vi "ESP32_Task_4.vi"() -> ()   [LabVIEW 2022 SP3]
doc: "This example performs writes and reads on a serial port, as directed by the user. You can press the Write and Read buttons, and change the Read Count, while the example is running.\n\nThe parameters set for the serial port must match the parameters of the connected instrument or device. In this example, the Read Count parameter specifies the number of bytes that the serial port reads. If there were more bytes at the port than the specified number, those bytes would not be read. If there were less bytes at the port than the specified number, you would receive a timeout error.\n\nThis example expands upon the flow control options for XON and XOFF, allowing the user to choose those control characters. Also, the user can enable or disable a termination character. Some devices require a termination character in order to identify the end of command strings. Some devices send a termination character to signify the end of data to be read. This example shows how you can end the Read operation once a termination character is detected in the buffer and/or append a termination character at the end of the Write data."
uses:
  Serial - Settings.ctl
  Serial - XON-XOFF Characters.ctl
  Serial - ASCII Characters.ctl
  ESP32-PSOC-State Machine.ctl
  <vilib>/Math Plots/2D Math Plots/2D Compass/2D Compass XCtrl/2D Compass.xctl
  <vilib>/Instr/_visa.llb/VISA Flush IO Buffer Mask.ctl
  <vilib>/Instr/_visa.llb/VISA Configure Serial Port (Instr).vi
  <vilib>/Math Plots/2D Math Plots/2D Compass/2D Compass Datatype/Public/Plot Helper (Vector).vi
  <vilib>/Math Plots/2D Math Plots/2D Compass/2D Compass Datatype/2D Compass Datatype.lvclass
panel:
  out "number 2":dbl
  out "number":dbl
  out "String":string
  out "XY Graph":cluster{"X":dbl, "Y":dbl}[](graph)
  out "2D Compass":refnum<class "2D Plot Datatype.lvclass">[](xcontrol)
  in  "Difficulty":T1
  out "error":bool
  out "Connected":bool
  out "Serial Settings:Number of Bytes at Serial Port":u32
  out "Response 2":string
  in  "Toggle LED":bool
  in  "Enum":T2
  in  "Termination Character":u8=10 format="%.0x"
  in  "End Write on Termination Character?":bool=TRUE
  in  "Stop":bool
  out "Read Count":u32=1000
  out "Response":string
  in  "XON/XOFF Characters":T3={"XON"=enum."DC1", "XOFF"=enum."DC3"}
  in  "Serial Settings":T5={"baud rate"=115200, "data bits"=8, "parity"=enum."None", "stop bits"=10, "flow control"=0} {"flow control" items=["None"=0, "XON/XOFF"=1, "RTS/CTS"=2, "DTR/DSR"=4]; "stop bits" items=["1.0"=10, "1.5"=15, "2.0"=20]; "data bits" min=5 max=8 step=1; "baud rate" items=["75"=75, "110"=110, "134"=134, "150"=150, "300"=300, "600"=600, "1200"=1200, "1800"=1800, "2400"=2400, "4800"=4800, "7200"=7200, "9600"=9600, "14400"=14400, "19200"=19200, "28800"=28800, "38400"=38400, "56000"=56000, "57600"=57600, "115200"=115200, "128000"=128000, "230400"=230400]}
  in  "End Read on Termination Character?":bool=TRUE
  in  "VISA resource name":refnum<visa-resource-name>="COM4"
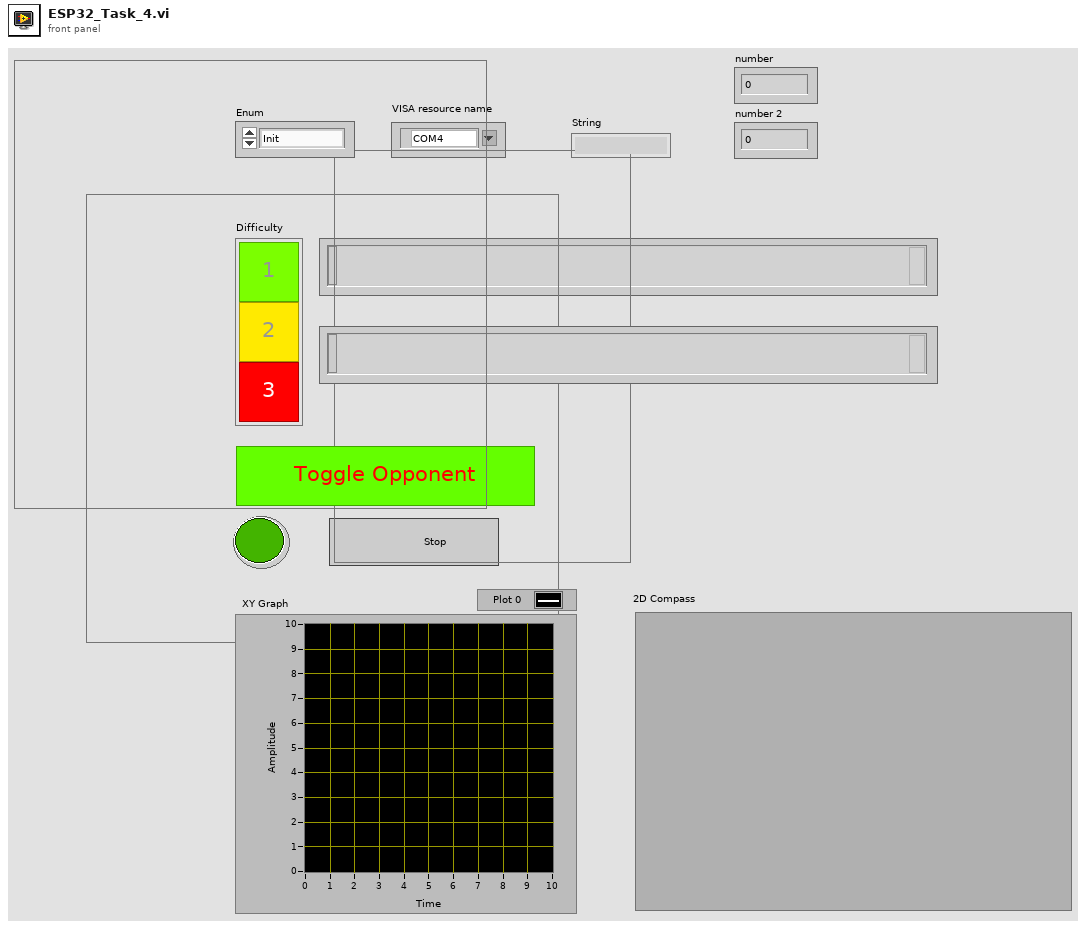
[diagram p1: front panel]
types:
  T1 = cluster{"Command A":bool, "Command B":bool, "Command C":bool}
  T2 = typedef "ESP32-PSOC-State Machine.ctl" = enum8{"Init", "Connect", "idle", "send", "wait", "receive", "que", "error", "exit"}
  T3 = typedef "Serial - XON-XOFF Characters.ctl" = cluster{"XON":T4, "XOFF":T4}
  T4 = typedef "Serial - ASCII Characters.ctl" = enum16{"NUL", "SOH", "STX", "ETX", "EOT", "ENQ", "ACK", "BEL", "BS", "HT", "LF", "VT", "FF", "CR", "SO", "SI", "DLE", "DC1", "DC2", "DC3", "DC4", "NAK", "SYN", "ETB", "CAN", "EM", "SUB", "ESC", "FS", "GS", "RS", "US", "SP", "!", "\"", "#", "$", "%", "&", "'", "(", ")", "*", "+", ",", "- (-)", ".", "/", "0", "1", "2", "3", "4", "5", "6", "7", "8", "9", ":", ";", "<", "=", ">", "?", "@", "A", "B", "C", "D", "E", "F", "G", "H", "I", "J", "K", "L", "M", "N", "O", "P", "Q", "R", "S", "T", "U", "V", "W", "X", "Y", "Z", "[", "\\", "]", "^", "_", "`", "a", "b", "c", "d", "e", "f", "g", "h", "i", "j", "k", "l", "m", "n", "o", "p", "q", "r", "s", "t", "u", "v", "w", "x", "y", "z", "{", "|", "}", "~"}
  T5 = typedef "Serial - Settings.ctl" = cluster{"baud rate":u32, "data bits":u16, "parity":enum16{"None", "Odd", "Even", "Mark", "Space"}, "stop bits":u16, "flow control":u16}
  T6 = typedef "VISA Flush IO Buffer Mask.ctl" = u16
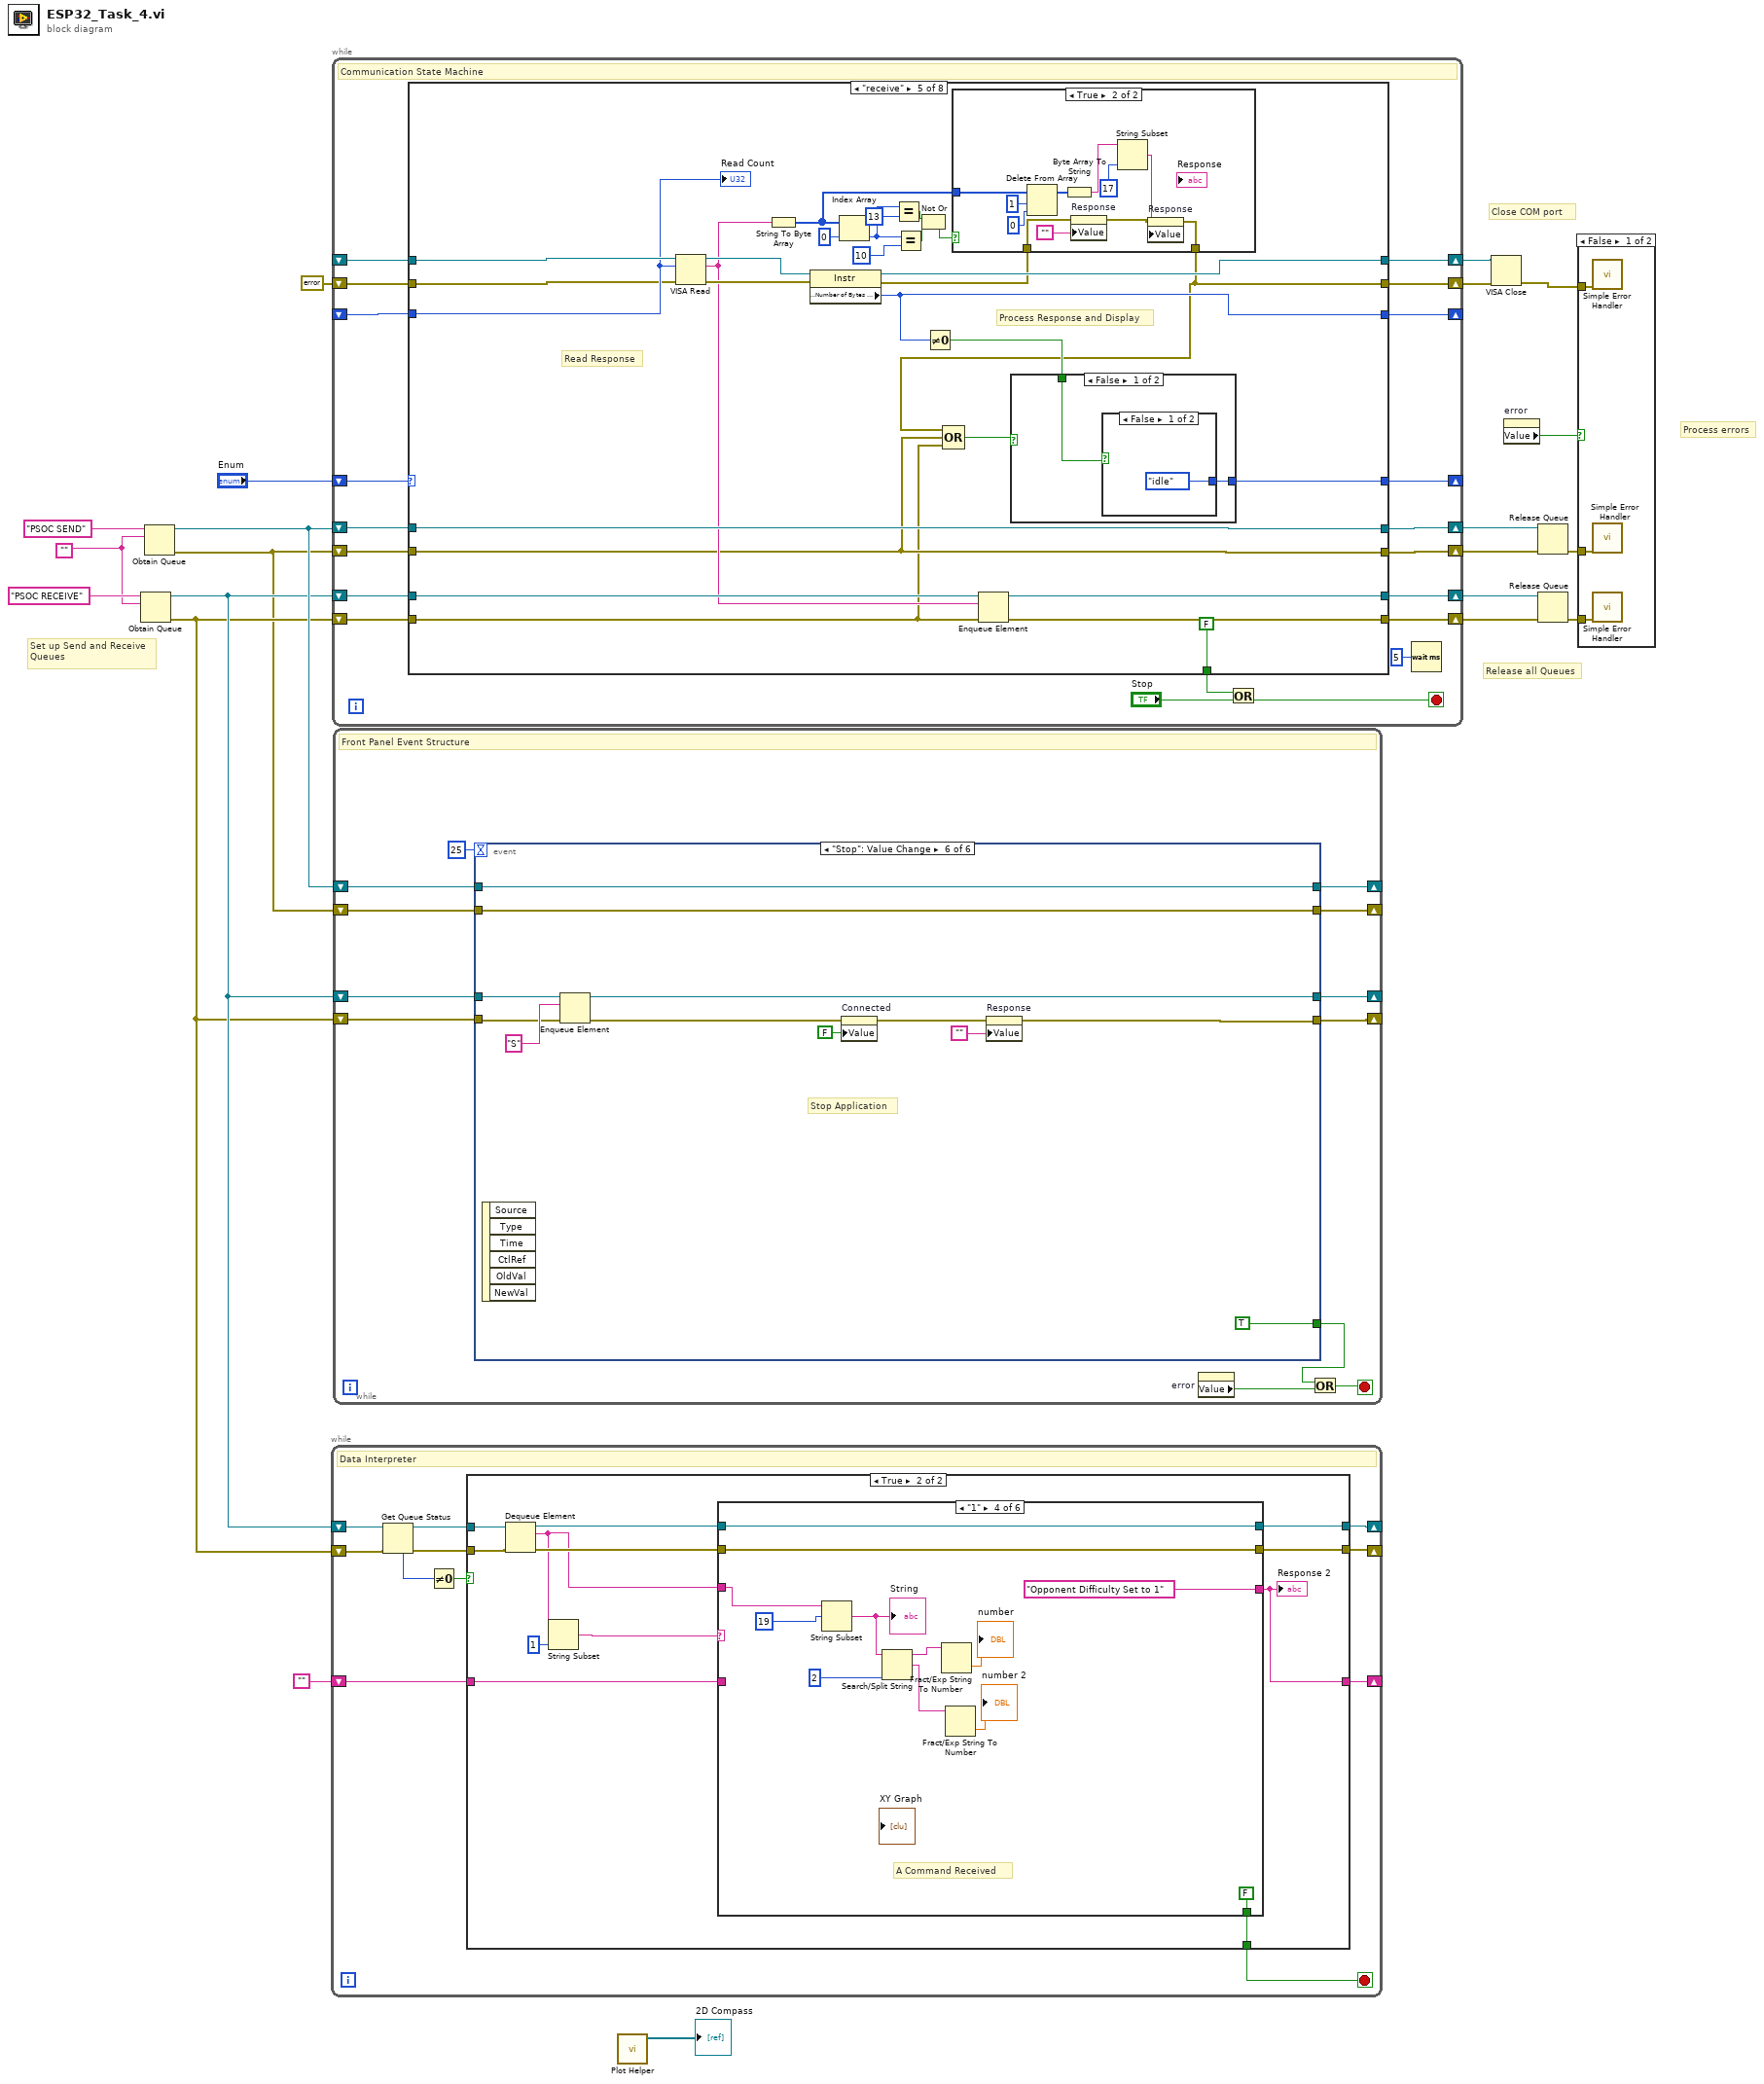
[diagram p0: block diagram]
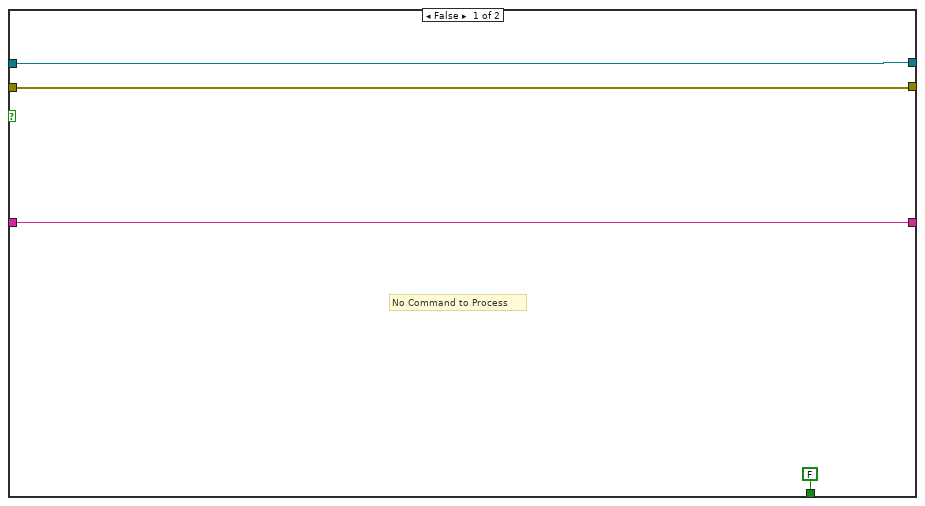
[diagram p3: hidden frame]
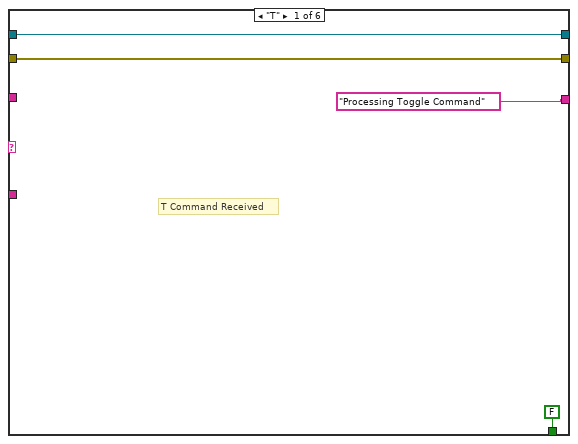
[diagram p4: hidden frame]
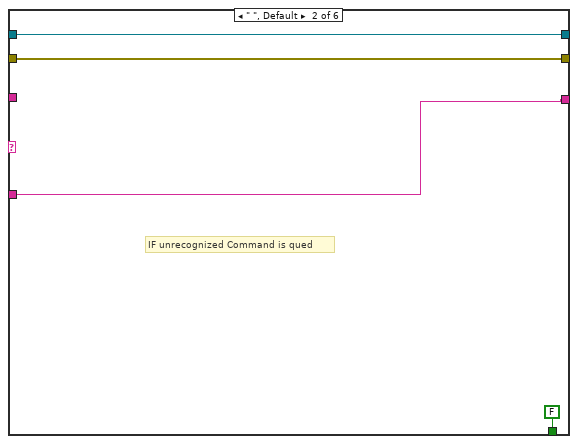
[diagram p5: hidden frame]
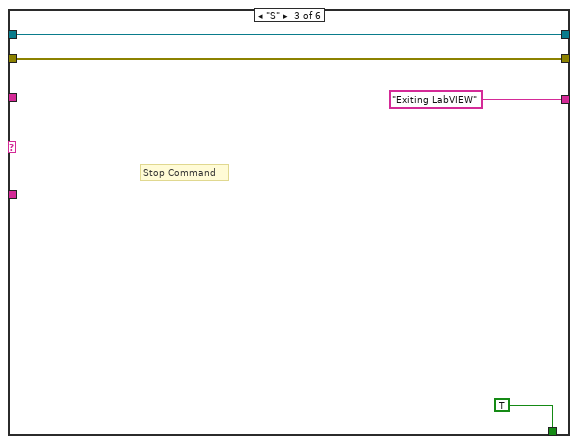
[diagram p6: hidden frame]
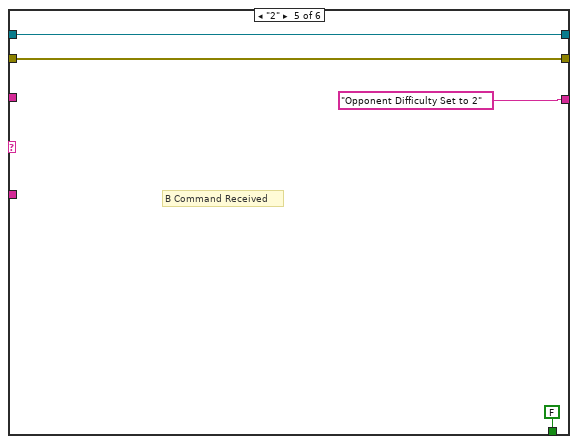
[diagram p7: hidden frame]
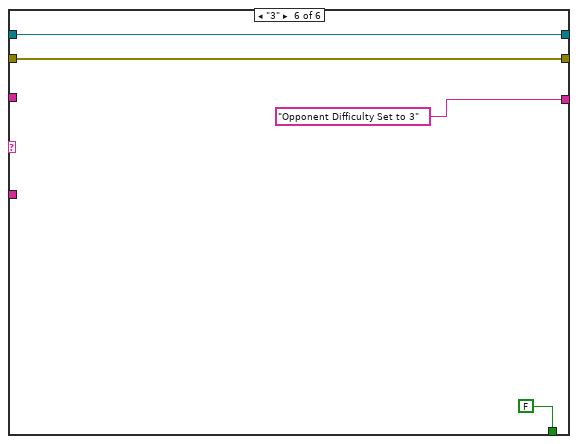
[diagram p8: hidden frame]
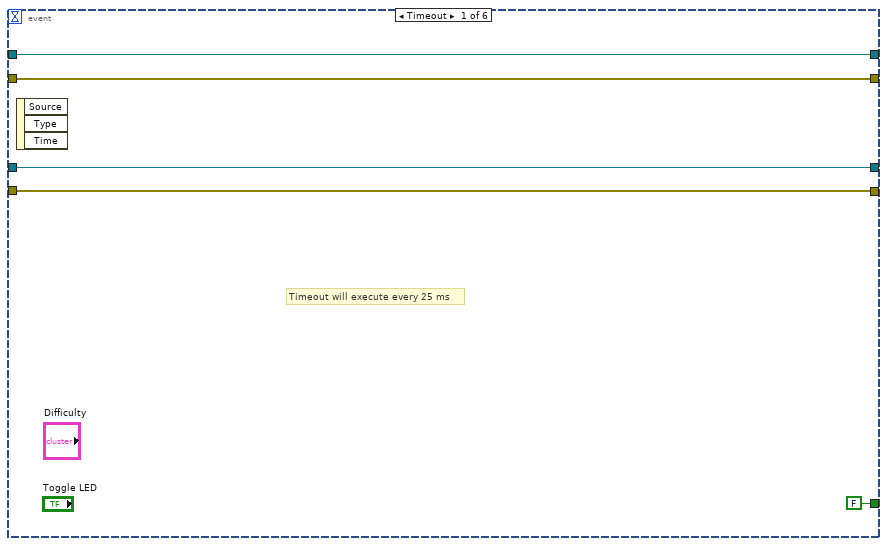
[diagram p9: hidden frame]
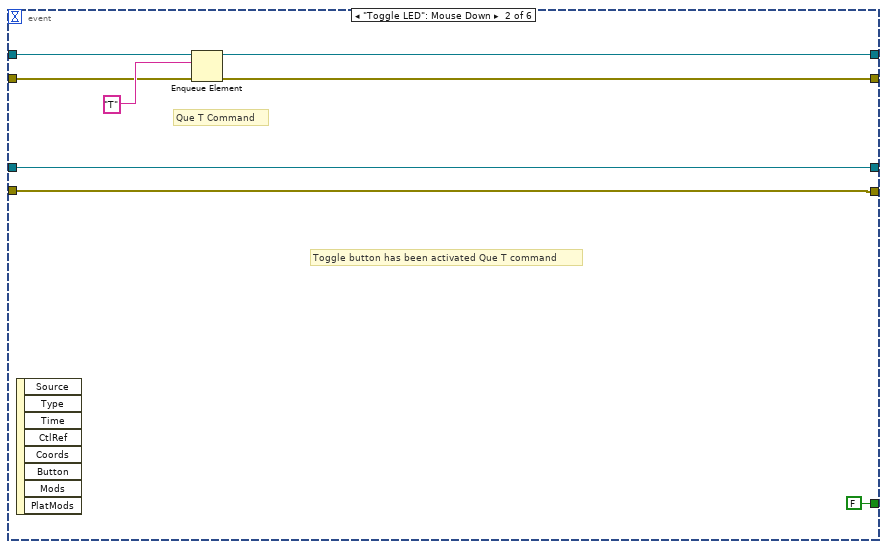
[diagram p10: hidden frame]
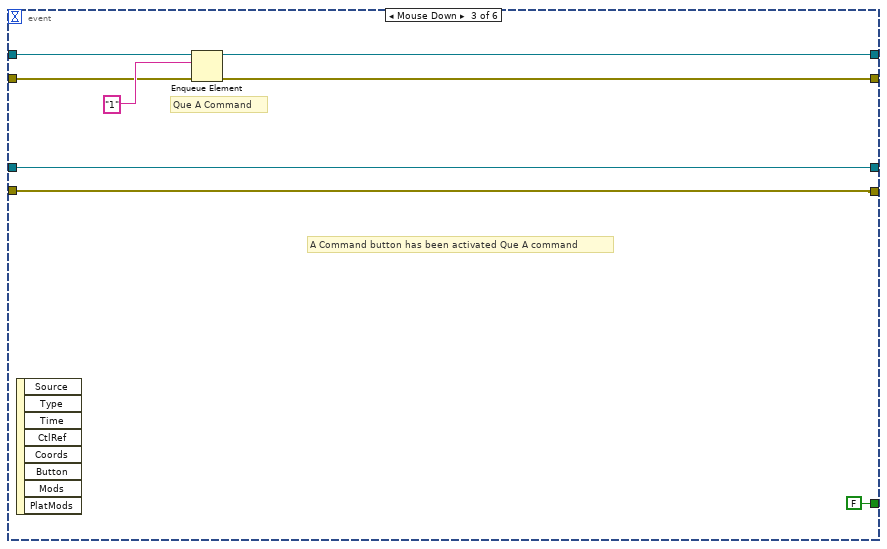
[diagram p11: hidden frame]
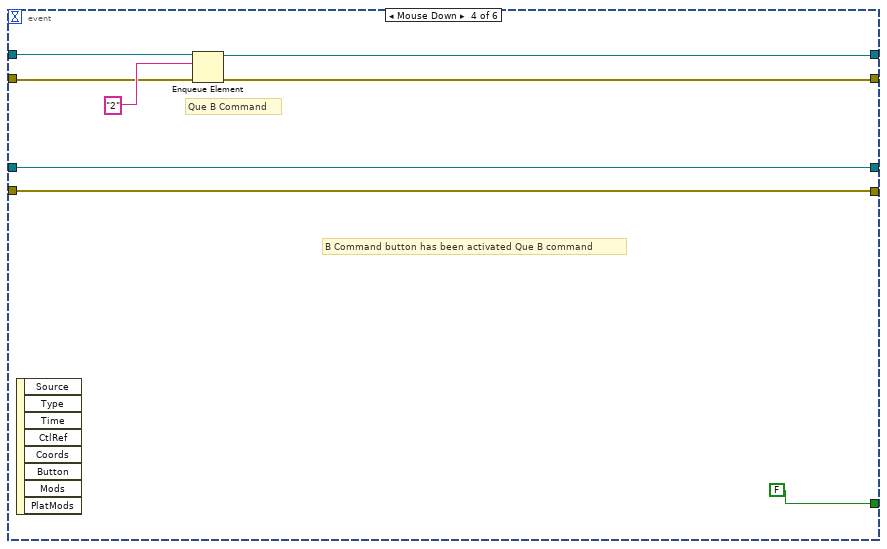
[diagram p12: hidden frame]
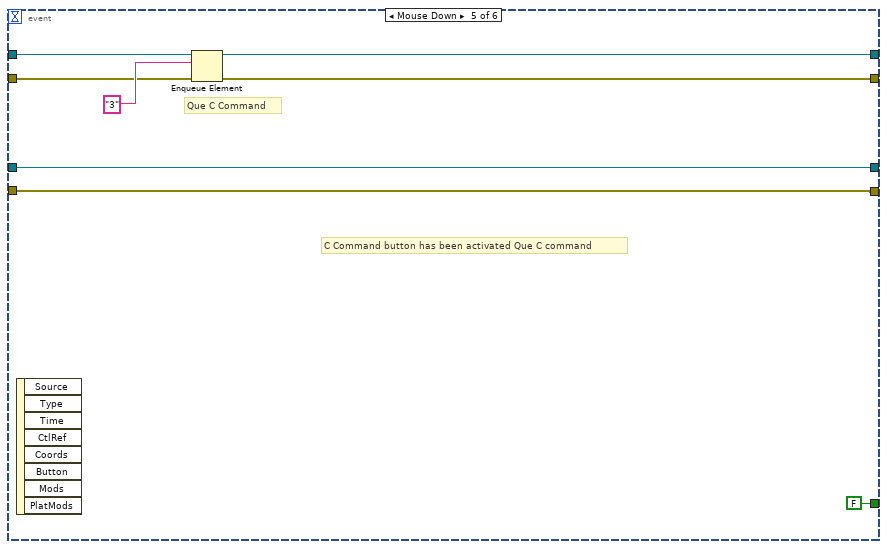
[diagram p13: hidden frame]
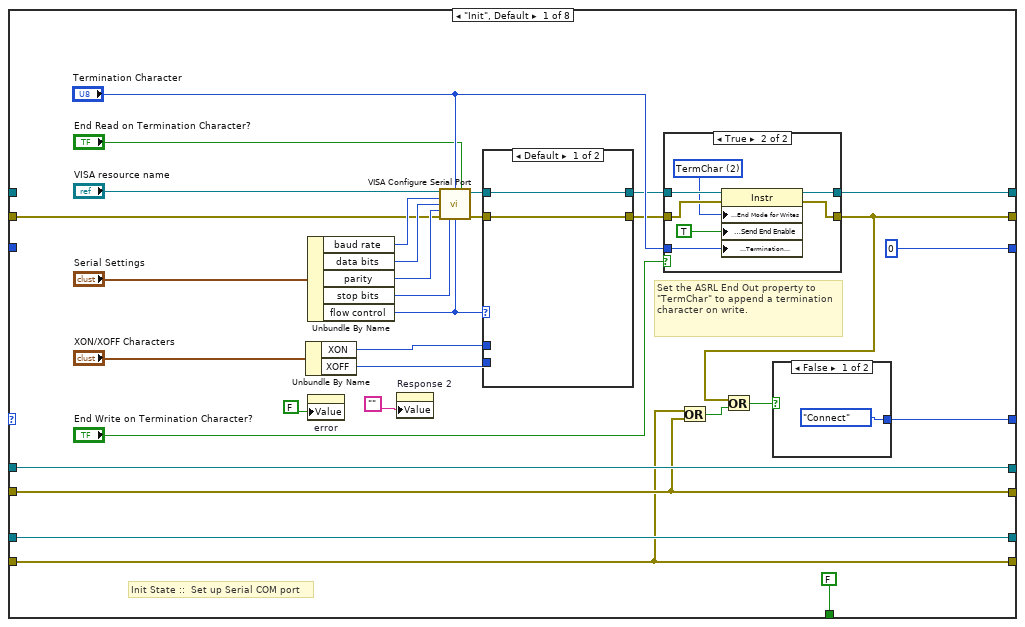
[diagram p14: hidden frame]
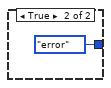
[diagram p15: hidden frame]
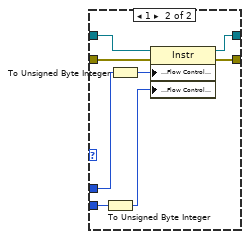
[diagram p17: hidden frame]
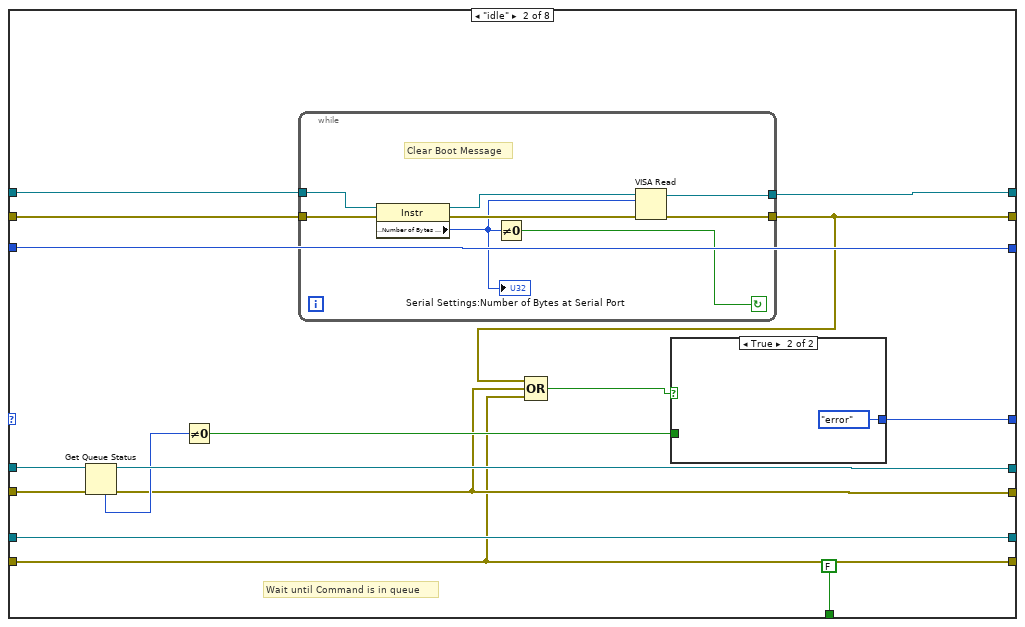
[diagram p18: hidden frame]
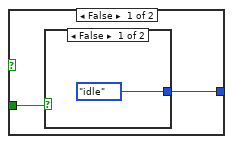
[diagram p19: hidden frame]
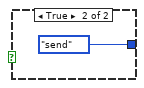
[diagram p20: hidden frame]
diagram:
  w11 = ""
  # "Process errors"
  # "Release all Queues"
  # "Close COM port"
  # "Set up Send and Receive\nQueues"
  n1 = Obtain Queue(name (unnamed)="PSOC RECEIVE", element data type=w11) -> (queue out=w10:refnum<queue>, error out=w9:errorcluster)  [unwired: 3 in, 1 out]
  n2 = Obtain Queue(name (unnamed)="PSOC SEND", element data type=w11) -> (queue out=w13:refnum<queue>, error out=w3:errorcluster)  [unwired: 3 in, 1 out]
  n3 = while {
    shift-right: [w26] -> _
    shift-left: w10 -> [w32]
    shift-right: [w25] -> _
    shift-left: w9 -> [w31]
    shift-right: [w23] -> _
    shift-left: "" -> [w22]
    stop <- w24 stop-if-true
    # "Data Interpreter"
    n4 = Get Queue Status(queue=w32, error in (no error)=w31) -> (queue out=w28:refnum<queue>, error out=w27:errorcluster, # elements in queue=w30:i32)  [unwired: 1 in, 5 out]
    n5 = Not Equal To 0?(x=w30) -> (x != 0?=w29:bool)
    n6 = case shown="True" w29 {
      tunnel: w28 -> [w36 w48]
      tunnel: w27 -> [w35 w41]
      tunnel: [w36 w46] -> w26
      tunnel: [w35 w45] -> w25
      tunnel: [FALSE w44] -> w24
      tunnel: [w33 w43] -> w23
      tunnel: w22 -> [w33 w42]
      frame False {
        # "No Command to Process"
      }
      frame True {
        n7 = Dequeue Element(queue=w48, error in (no error)=w41) -> (queue out=w39:refnum<queue>, element=w38:string, error out=w40:errorcluster)  [unwired: 1 in, 1 out]
        n8 = String Subset(string=w38, length (rest)=1 ("length (rest)")) -> (substring=w37:string)  [unwired: 1 in]
        n9 = case shown="\"1\"" w37 {
          tunnel: w39 -> [w52 w56 w60 w69 w76 w79]
          tunnel: w40 -> [w51 w55 w59 w72 w75 w78]
          tunnel: [w52 w56 w60 w69 w76 w79] -> w46
          tunnel: [w51 w55 w59 w72 w75 w78] -> w45
          tunnel: w38 -> [_ _ _ w68 _ _]
          tunnel: [FALSE FALSE TRUE FALSE FALSE FALSE] -> w44
          tunnel: ["Processing Toggle Command" w53 "Exiting LabVIEW" "Opponent Difficulty Set to 1" "Opponent Difficulty Set to 2" "Opponent Difficulty Set to 3"] -> w43
          tunnel: w42 -> [_ w53 _ _ _ _]
          frame "T" {
            # "T Command Received"
          }
          frame " ", Default {
            # "IF unrecognized Command is qued"
          }
          frame "S" {
            # "Stop Command"
          }
          frame "1" {
            # "A Command Received"
            n10 = String Subset(string=w68, offset (0)=19 ("length (rest)")) -> (substring=w65:string)  [unwired: 1 in]
            "String" <- w65
            n11 = Search/Split String(string=w65, offset (0)=2 ("length (rest)")) -> (substring before match=w61:string, match + rest of string=w62:string)  [unwired: 1 in, 1 out]
            n12 = Fract/Exp String To Number(string=w61) -> (number=→"number":dbl)  [unwired: 3 in, 1 out]
            n13 = Fract/Exp String To Number(string=w62) -> (number=→"number 2":dbl)  [unwired: 3 in, 1 out]
          }
          frame "2" {
            # "B Command Received"
          }
          frame "3" {
          }
        }
        "Response 2" <- w43
      }
    }
  }
  n14 = while {
    shift-right: [w92] -> w21
    shift-left: w13 -> [w100]
    shift-right: [w91] -> w19
    shift-left: w3 -> [w99]
    shift-right: [w90] -> w20
    shift-left: w10 -> [w98]
    shift-right: [w89] -> w16
    shift-left: w9 -> [w97]
    shift-right: [w84] -> _
    shift-left: "Enum" -> [w83]
    shift-right: [w96] -> w15
    shift-left: _ -> [w93]
    shift-right: [w95] -> w14
    shift-left: errorcluster {"status"=FALSE, "code"=0, "source"=""} ("error out") -> [w94]
    shift-right: [w88] -> _
    shift-left: _ -> [w87]
    stop <- w82 stop-if-true
    # "Communication State Machine"
    n15 = case shown="\"receive\"" w83 {
      selector: w83 -> [_ _ _ _ _ _ w302 _]
      tunnel: [w130 w166 w205 w222 w259 w286 w301 w324] -> w92
      tunnel: [w104 w156 w196 w216 w241 w283 w300 w323] -> w91
      tunnel: [w110 w164 w197 w225 w260 ESP32-PSOC-State_Machine."exit" ("Enum") w302 ESP32-PSOC-State_Machine."idle" ("Enum")] -> w84
      tunnel: w100 -> [w130 w168 w207 w222 w259 w286 w301 w324]
      tunnel: w99 -> [w104 w167 w206 w216 w241 w283 w300 w323]
      tunnel: w98 -> [w131 w162 w204 w219 w254 w285 w299 w322]
      tunnel: w97 -> [w103 w155 w195 w215 w240 w282 w290 w321]
      tunnel: [w112 w159 w191 w224 w249 w288 w305 w326] -> w96
      tunnel: [w106 w157 w192 w217 w242 w284 w304 w327] -> w95
      tunnel: w94 -> [w108 w158 w200 w223 w244 w284 w304 w328]
      tunnel: w93 -> [_ w160 w202 w213 w257 w288 w305 w329]
      tunnel: [w131 w162 w204 w219 w252 w285 w297 w322] -> w90
      tunnel: [w103 w155 w195 w215 w253 w282 w293 w321] -> w89
      tunnel: [u32 0 ("Bytes at Port") w161 w203 w221 w255 w287 w303 w325] -> w88
      tunnel: w87 -> [_ w161 w203 _ w251 w287 w303 w325]
      tunnel: [FALSE FALSE FALSE FALSE FALSE FALSE TRUE FALSE] -> w81
      frame "Init", Default {
        # "Init State ::  Set up Serial COM port"
        # "Set the ASRL End Out property to \"TermChar\" to append a termination character on write."
        n16 = Unbundle By Name("XON/XOFF Characters") -> ("XON"=w124:T4, "XOFF"=w125:T4)
        n17 = Unbundle By Name("Serial Settings") -> ("baud rate"=w120:u32, "data bits"=w119:u16, "parity"=w118:enum16{"None", "Odd", "Even", "Mark", "Space"}, "stop bits"=w117:u16, "flow control"=w123:u16)
        n18 = property on="error" class="Bool (strict)"("Value"=FALSE ("error")) -> ()  [unwired: 2 in, 2 out]
        n19 = property on="Response 2" class="Str"("Value"="") -> ()  [unwired: 2 in, 2 out]
        n20 = call-poly "VISA Configure Serial Port"("VISA resource name"="VISA resource name", "termination char\n(0xA = '\\n' = LF)"="Termination Character", "Enable Termination\nChar (T)"="End Read on Termination Character?", "baud rate (9600)"=w120, "data bits (8)"=w119, "parity (0:none)"=w118, "error in (no error)"=w108, "stop bits (10: 1 bit)"=w117, "flow control (0:none)"=w123) -> ("VISA resource name out"=w116:refnum<visa-resource-name>, "error out"=w115:errorcluster)  [unwired: 1 in, 4 out]
        n21 = case shown="Default" w123 {
          tunnel: [w143 w152] -> w126
          tunnel: [w144 w151] -> w127
          tunnel: w115 -> [w143 w150]
          tunnel: w116 -> [w144 w149]
          tunnel: w124 -> [_ w148]
          tunnel: w125 -> [_ w147]
          frame Default {
          }
          frame 1 {
            n22 = To Unsigned Byte Integer(number=w147) -> (unsigned 8bit integer=w146:u8)
            n23 = To Unsigned Byte Integer(number=w148) -> (unsigned 8bit integer=w145:u8)
            n24 = property class="Instr"(reference=w149, error in=w150, "Serial Settings:Flow Control XON Character"=w145, "Serial Settings:Flow Control XOFF Character"=w146) -> (reference out=w151:refnum<visa-resource-name>, error out=w152:errorcluster)
          }
        }
        n25 = case shown="True" "End Write on Termination Character?" {
          tunnel: w127 -> [w134 w142]
          tunnel: w126 -> [w135 w141]
          tunnel: [w134 w140] -> w112
          tunnel: [w135 w139] -> w106
          tunnel: "Termination Character" -> [_ w137]
          frame False {
          }
          frame True {
            w138 = u16 2 items=["None", "LastBit", "TermChar", "Break"] ("Serial Settings:Serial End Mode for Writes")
            n26 = property class="Instr"(reference=w142, error in=w141, "Serial Settings:End Mode for Writes"=w138, "Message Based Settings:Send End Enable"=TRUE, "Message Based Settings:Termination Character"=w137) -> (reference out=w140:refnum<visa-resource-name>, error out=w139:errorcluster)
          }
        }
        n27 = Or(x=w103, y=w104) -> (x .or. y?=w105:bool)
        n28 = Or(x=w106, y=w105) -> (x .or. y?=w107:bool)
        n29 = case shown="False" w107 {
          tunnel: [ESP32-PSOC-State_Machine."Connect" ("Enum") ESP32-PSOC-State_Machine."error" ("Enum")] -> w110
          frame False {
          }
          frame True {
          }
        }
      }
      frame "idle" {
        # "Wait until Command is in queue"
        n30 = Get Queue Status(queue=w168, error in (no error)=w167) -> (queue out=w166:refnum<queue>, error out=w156:errorcluster, # elements in queue=w165:i32)  [unwired: 1 in, 5 out]
        n31 = Not Equal To 0?(x=w165) -> (x != 0?=w163:bool)
        n32 = while {
          tunnel: w160 -> [w181]
          tunnel: [w177] -> w159
          tunnel: w158 -> [w180]
          tunnel: [w175] -> w157
          stop <- w179 continue-if-true
          # "Clear Boot Message"
          n33 = property class="Instr"(reference=w181, error in=w180) -> (reference out=w178:refnum<visa-resource-name>, error out=w176:errorcluster, "Serial Settings:Number of Bytes at Serial Port"=w174:u32)
          "Serial Settings:Number of Bytes at Serial Port" <- w174
          n34 = Not Equal To 0?(x=w174) -> (x != 0?=w179:bool)
          n35 = VISA Read(VISA resource name=w178, byte count=w174, error in (no error)=w176) -> (VISA resource name out=w177:refnum<visa-resource-name>, error out=w175:errorcluster)  [unwired: 2 out]
        }
        n36 = Compound Arithmetic op=OR(w157, w156, w155) -> (w154:bool)
        n37 = case shown="True" w154 {
          tunnel: [w170 ESP32-PSOC-State_Machine."error" ("Enum")] -> w164
          tunnel: w163 -> [w169 _]
          frame False {
            n38 = case shown="False" w169 {
              tunnel: [ESP32-PSOC-State_Machine."idle" ("Enum") ESP32-PSOC-State_Machine."send" ("Enum")] -> w170
              frame False {
              }
              frame True {
              }
            }
          }
          frame True {
          }
        }
      }
      frame "send" {
        w198 = T6 64 items=["Flush Receive Buffer"=16, "Write Transmit Buffer to Device"=32, "Flush Receive Buffer (No I/O)"=64, "Flush Transmit Buffer"=128] ("Mask")
        # "Read and Discard Echo Command"
        # "Wait for Response"
        # "Send Command"
        n39 = Dequeue Element(queue=w207, error in (no error)=w206) -> (queue out=w205:refnum<queue>, element=w185:string, error out=w196:errorcluster)  [unwired: 1 in, 1 out]
        n40 = VISA Flush I/O Buffer(VISA resource name=w202, mask (16)=w198, error in (no error)=w200) -> (VISA resource name out=w201:refnum<visa-resource-name>, error out=w199:errorcluster)
        n41 = Concatenate Strings(w185, "\r\n") -> (w184:string)
        n42 = VISA Write(VISA resource name=w201, write buffer=w184, error in (no error)=w199) -> (VISA resource name out=w183:refnum<visa-resource-name>, error out=w189:errorcluster)  [unwired: 1 out]
        n43 = flat-sequence {
          tunnel: w183 -> [w209]
          tunnel: [w209] -> w182
          frame #0 {
            n44 = Wait (ms)(milliseconds to wait=u32 15) -> ()  [unwired: 1 out]
          }
        }
        n45 = property class="Instr"(reference=w182, error in=w189) -> (reference out=w190:refnum<visa-resource-name>, error out=w188:errorcluster, "Serial Settings:Number of Bytes at Serial Port"=w187:u32)
        n46 = VISA Read(VISA resource name=w190, byte count=w187, error in (no error)=w188) -> (VISA resource name out=w191:refnum<visa-resource-name>, error out=w192:errorcluster)  [unwired: 2 out]
        n47 = Compound Arithmetic op=OR(w192, w196, w195) -> (w194:bool)
        n48 = case shown="False" w194 {
          tunnel: [ESP32-PSOC-State_Machine."wait" ("Enum") ESP32-PSOC-State_Machine."error" ("Enum")] -> w197
          frame False {
          }
          frame True {
          }
        }
      }
      frame "wait" {
        # "Wait for actual Response"
        n49 = flat-sequence {
          tunnel: w213 -> [w227]
          tunnel: [w227] -> w212
          frame #0 {
            n50 = Wait (ms)(milliseconds to wait=u32 15) -> ()  [unwired: 1 out]
          }
        }
        n51 = property class="Instr"(reference=w212, error in=w223) -> (reference out=w224:refnum<visa-resource-name>, error out=w217:errorcluster, "Serial Settings:Number of Bytes at Serial Port"=w221:u32)
        n52 = Not Equal To 0?(x=w221) -> (x != 0?=w220:bool)
        n53 = Compound Arithmetic op=OR(w217, w216, w215) -> (w218:bool)
        n54 = case shown="False" w218 {
          tunnel: [w229 ESP32-PSOC-State_Machine."error" ("Enum")] -> w225
          tunnel: w220 -> [w228 _]
          frame False {
            n55 = case shown="True" w228 {
              tunnel: [ESP32-PSOC-State_Machine."wait" ("Enum") ESP32-PSOC-State_Machine."receive" ("Enum")] -> w229
              frame False {
              }
              frame True {
              }
            }
          }
          frame True {
          }
        }
      }
      frame "receive" {
        # "Process Response and Display"
        # "Read Response"
        n56 = VISA Read(VISA resource name=w257, byte count=w251, error in (no error)=w244) -> (VISA resource name out=w250:refnum<visa-resource-name>, read buffer=w246:string, error out=w256:errorcluster)  [unwired: 1 out]
        n57 = String To Byte Array(string=w246) -> (unsigned byte array=w245:u8[])
        n58 = property class="Instr"(reference=w250, error in=w256) -> (reference out=w249:refnum<visa-resource-name>, error out=w243:errorcluster, "Serial Settings:Number of Bytes at Serial Port"=w255:u32)
        n59 = Index Array(array=w245, index=0) -> (element=w237:u8)
        n60 = Equal?(x=w237, y=u8 13) -> (x = y?=w235:bool)
        n61 = Equal?(x=w237, y=u8 10) -> (x = y?=w234:bool)
        n62 = Not Or(1:w234, 2:w235) -> (0:w233:bool)
        n63 = Not Equal To 0?(x=w255) -> (x != 0?=w258:bool)
        n64 = case shown="True" w233 {
          tunnel: w245 -> [_ w277]
          tunnel: w243 -> [w266 w271]
          tunnel: [w266 w270] -> w242
          frame False {
          }
          frame True {
            n65 = Delete From Array(array=w277, length=1, index=0) -> (array with subset deleted=w274:u8[])  [unwired: 1 out]
            n66 = Byte Array To String(unsigned byte array=w274) -> (string=w269:string)
            n67 = property on="Response" class="Str"(error in=w271, "Value"="") -> (error out=w272:errorcluster)  [unwired: 1 in, 1 out]
            n68 = String Subset(string=w269, length (rest)=17 ("length")) -> (substring=w268:string)  [unwired: 1 in]
            n69 = property on="Response" class="Str"(error in=w272, "Value"=w268) -> (error out=w270:errorcluster)  [unwired: 1 in, 1 out]
          }
        }
        n70 = Compound Arithmetic op=OR(w242, w241, w240) -> (w239:bool)
        n71 = Enqueue Element(queue=w254, element=w246, error in (no error)=w240) -> (queue out=w252:refnum<queue>, error out=w253:errorcluster)  [unwired: 1 in, 1 out]
        n72 = case shown="False" w239 {
          tunnel: [w262 ESP32-PSOC-State_Machine."error" ("Enum")] -> w260
          tunnel: w258 -> [w261 _]
          frame False {
            n73 = case shown="False" w261 {
              tunnel: [ESP32-PSOC-State_Machine."idle" ("Enum") ESP32-PSOC-State_Machine."receive" ("Enum")] -> w262
              frame False {
              }
              frame True {
              }
            }
          }
          frame True {
          }
        }
        "Read Count" <- w251
      }
      frame "error" {
        # "Process any error"
        n74 = Build Array(w284, w283, w282) -> (w281:errorcluster[])
        n75 = for {
          tunnel: w281 -> [w289] mode=indexing
          n76 = call <vilib>:"General Error Handler.vi"("error in (no error)"=w289) -> ()  [unwired: 10 in, 5 out]
        }
        "error" <- TRUE ("error")
      }
      frame "exit" {
        # "Exit due to error"
        n77 = Enqueue Element(queue=w299, element="S", error in (no error)=w290) -> (queue out=w297:refnum<queue>, error out=w295:errorcluster)  [unwired: 1 in, 1 out]
        n78 = property on="Connected" class="Bool (strict)"(error in=w295, "Value"=FALSE ("Connected")) -> (error out=w294:errorcluster)  [unwired: 1 in, 1 out]
        n79 = property on="Response" class="Str"(error in=w294, "Value"="") -> (error out=w293:errorcluster)  [unwired: 1 in, 1 out]
      }
      frame "Connect" {
        # "Validating connection"
        # "Send ID to validate connection"
        # "Clear any residual characters"
        n80 = while {
          shift-right: [w353] -> w317
          shift-left: w328 -> [w359]
          shift-right: [w352] -> w318
          shift-left: w329 -> [w358]
          stop <- w357 continue-if-true
          n81 = property class="Instr"(reference=w358, error in=w359) -> (reference out=w355:refnum<visa-resource-name>, error out=w354:errorcluster, "Bytes at Port"=w351:u32)
          n82 = VISA Read(VISA resource name=w355, byte count=w351, error in (no error)=w354) -> (VISA resource name out=w352:refnum<visa-resource-name>, read buffer=w350:string, error out=w353:errorcluster)  [unwired: 1 out]
          n83 = Wait (ms)(milliseconds to wait=u32 5) -> ()  [unwired: 1 out]
          n84 = Search/Split String(string=w350, search string/char (-)="Commands") -> (match + rest of string=w348:string)  [unwired: 1 in, 2 out]
          n85 = String Length(string=w348) -> (length=w347:i32)
          n86 = Equal To 0?(x=w347) -> (x = 0?=w357:bool)
        }
        n87 = Concatenate Strings("I" ("write buffer"), "\r\n") -> (w306:string)
        n88 = VISA Write(VISA resource name=w318, write buffer=w306, error in (no error)=w317) -> (VISA resource name out=w312:refnum<visa-resource-name>, error out=w316:errorcluster)  [unwired: 1 out]
        n89 = flat-sequence {
          tunnel: w312 -> [w346]
          tunnel: [w346] -> w311
          frame #0 {
            n90 = Wait (ms)(milliseconds to wait=u32 5) -> ()  [unwired: 1 out]
          }
        }
        n91 = property class="Instr"(reference=w311, error in=w316) -> (reference out=w314:refnum<visa-resource-name>, error out=w315:errorcluster, "Bytes at Port"=w313:u32)
        n92 = VISA Read(VISA resource name=w314, byte count=w313, error in (no error)=w315) -> (VISA resource name out=w309:refnum<visa-resource-name>, error out=w310:errorcluster)  [unwired: 2 out]
        n93 = while {
          shift-right: [w333] -> w327
          shift-left: w310 -> [w339]
          shift-right: [w334] -> w326
          shift-left: w309 -> [w332]
          stop <- w330 stop-if-true
          n94 = flat-sequence {
            tunnel: w332 -> [w344]
            tunnel: [w344] -> w331
            frame #0 {
              n95 = Wait (ms)(milliseconds to wait=u32 15) -> ()  [unwired: 1 out]
            }
          }
          n96 = property class="Instr"(reference=w331, error in=w339) -> (reference out=w337:refnum<visa-resource-name>, error out=w338:errorcluster, "Bytes at Port"=w336:u32)
          n97 = VISA Read(VISA resource name=w337, byte count=w336, error in (no error)=w338) -> (VISA resource name out=w334:refnum<visa-resource-name>, read buffer=w335:string, error out=w333:errorcluster)  [unwired: 1 out]
          n98 = Search/Split String(string=w335, search string/char (-)="IESP32") -> (match + rest of string=w341:string)  [unwired: 1 in, 2 out]
          n99 = String Length(string=w341) -> (length=w340:i32)
          n100 = Not Equal To 0?(x=w340) -> (x != 0?=w330:bool)
          "Connected" <- w330
        }
      }
    }
    n101 = Or(x=w81, y="Stop") -> (x .or. y?=w82:bool)
    n102 = Wait (ms)(milliseconds to wait=u32 5) -> ()  [unwired: 1 out]
  }
  n103 = while {
    shift-right: [w368] -> _
    shift-left: w13 -> [w369]
    shift-right: [w367] -> _
    shift-left: w3 -> [w370]
    shift-right: [w363] -> _
    shift-left: w10 -> [w366]
    shift-right: [w364] -> _
    shift-left: w9 -> [w365]
    stop <- w360 stop-if-true
    # "Front Panel Event Structure"
    n104 = event shown="[5] \"Stop\": Value Change" {
      selector: _ -> [_ _ _ _ _ _]
      dyn-events: _ -> [_ _ _ _ _ _]
      timeout: 25 -> [_ _ _ _ _ _]
      tunnel: w370 -> [w374 w382 w390 w396 w406 w418]
      tunnel: w369 -> [w375 w384 w392 w397 w408 w419]
      tunnel: [w375 w381 w389 w399 w405 w419] -> w368
      tunnel: [w374 w380 w388 w398 w404 w418] -> w367
      tunnel: [FALSE FALSE FALSE FALSE FALSE TRUE] -> w362
      tunnel: w366 -> [w373 w378 w386 w395 w402 w417]
      tunnel: w365 -> [w372 w377 w385 w394 w401 w415]
      tunnel: [w372 w377 w385 w394 w401 w410] -> w364
      tunnel: [w373 w378 w386 w395 w402 w414] -> w363
      event Timeout {
        # "Timeout will execute every 25 ms"
        n105 = event-data() -> ()  [unwired: 1 in, 3 out]
      }
      event "Toggle LED": Mouse Down {
        # "Que T Command"
        # "Toggle button has been activated Que T command"
        n106 = event-data() -> ()  [unwired: 1 in, 8 out]
        n107 = Enqueue Element(queue=w384, element="T", error in (no error)=w382) -> (queue out=w381:refnum<queue>, error out=w380:errorcluster)  [unwired: 1 in, 1 out]
      }
      event "Difficulty.Command A": Mouse Down {
        # "Que A Command"
        # "A Command button has been activated Que A command"
        n108 = event-data() -> ()  [unwired: 1 in, 8 out]
        n109 = Enqueue Element(queue=w392, element="1", error in (no error)=w390) -> (queue out=w389:refnum<queue>, error out=w388:errorcluster)  [unwired: 1 in, 1 out]
      }
      event "Difficulty.Command B": Mouse Down {
        # "Que B Command"
        # "B Command button has been activated Que B command"
        n110 = event-data() -> ()  [unwired: 1 in, 8 out]
        n111 = Enqueue Element(queue=w397, element="2", error in (no error)=w396) -> (queue out=w399:refnum<queue>, error out=w398:errorcluster)  [unwired: 1 in, 1 out]
      }
      event "Difficulty.Command C": Mouse Down {
        # "Que C Command"
        # "C Command button has been activated Que C command"
        n112 = event-data() -> ()  [unwired: 1 in, 8 out]
        n113 = Enqueue Element(queue=w408, element="3", error in (no error)=w406) -> (queue out=w405:refnum<queue>, error out=w404:errorcluster)  [unwired: 1 in, 1 out]
      }
      event "Stop": Value Change {
        # "Stop Application"
        n114 = event-data() -> ()  [unwired: 1 in, 6 out]
        n115 = Enqueue Element(queue=w417, element="S", error in (no error)=w415) -> (queue out=w414:refnum<queue>, error out=w413:errorcluster)  [unwired: 1 in, 1 out]
        n116 = property on="Connected" class="Bool (strict)"(error in=w413, "Value"=FALSE ("Connected")) -> (error out=w411:errorcluster)  [unwired: 1 in, 1 out]
        n117 = property on="Response" class="Str"(error in=w411, "Value"="") -> (error out=w410:errorcluster)  [unwired: 1 in, 1 out]
      }
    }
    n118 = property on="error" class="Bool (strict)"() -> ("Value"=w361:bool)  [unwired: 2 in, 2 out]
    n119 = Or(x=w362, y=w361) -> (x .or. y?=w360:bool)
  }
  n120 = call-poly <vilib>:"Plot Helper.vi"() -> ("2D Plot Class Obj Array out"=→"2D Compass":refnum<class "2D Plot Datatype.lvclass">[])  [unwired: 4 in, 7 out]
  n121 = VISA Close(VISA resource name=w15, error in (no error)=w14) -> (error out=w6:errorcluster)
  n122 = property on="error" class="Bool (strict)"() -> ("Value"=w2:bool)  [unwired: 2 in, 2 out]
  n123 = Release Queue(queue=w21, error in (no error)=w19) -> (error out=w5:errorcluster)  [unwired: 1 in, 2 out]
  n124 = Release Queue(queue=w20, error in (no error)=w16) -> (error out=w4:errorcluster)  [unwired: 1 in, 2 out]
  n125 = case shown="False" w2 {
    tunnel: w6 -> [w423 _]
    tunnel: w5 -> [w422 _]
    tunnel: w4 -> [w421 _]
    frame False {
      n126 = call <vilib>:"Simple Error Handler.vi"("error in (no error)"=w423) -> ()  [unwired: 1 in, 8 out]
      n127 = call <vilib>:"Simple Error Handler.vi"("error in (no error)"=w422) -> ()  [unwired: 1 in, 8 out]
      n128 = call <vilib>:"Simple Error Handler.vi"("error in (no error)"=w421) -> ()  [unwired: 1 in, 8 out]
    }
    frame True {
    }
  }
